vi "Image scale.vi"(2 "Error in":errorcluster, 3 "Scale factor":dbl=1.0, 4 "Image in":T1) -> (0 "Error Out":errorcluster, 1 "Image Out":T1)   [LabVIEW 2014]
uses:
  <vilib>/vision/Image Controls.llb/IMAQ Image.ctl
  <vilib>/vision/NI_Vision_Development_Module.lvlib
panel:
  # "Paul Nathan 10/06/2015"
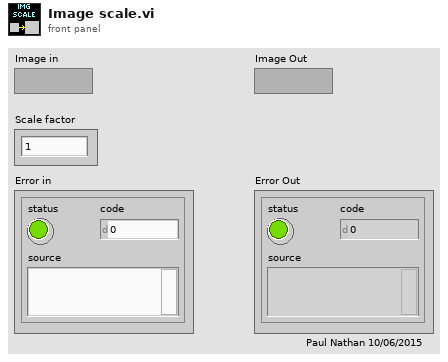
[diagram p1: front panel]
types:
  T1 = typedef "IMAQ Image.ctl" = refnum<image>
  T2 = cluster{"Red (or Hue) value":u8, "Green (or Sat) value":u8, "Blue (or Light or Val) value":u8}[][]
  T3 = cluster{"Red or Hue value":u8, "Green or Sat value":u8, "Blue or Luma or Val or Inten value":u8}
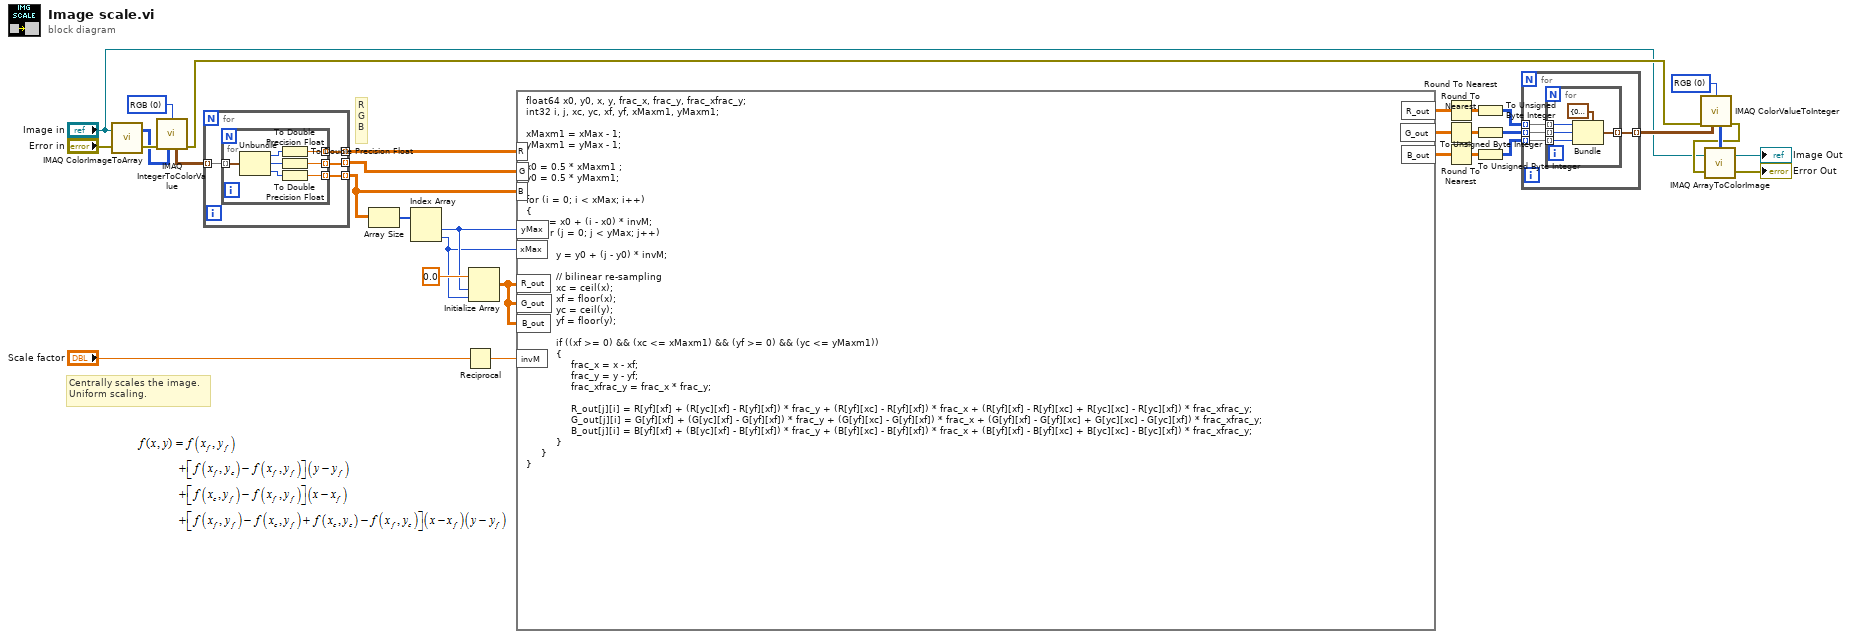
[diagram p0: block diagram]
diagram:
  w11 = u16 0 items=["RGB", "HSL", "HSV", "HSI"] ("Color Mode")
  w29 = u16 0 items=["RGB", "HSL", "HSV", "HSI"] ("Color Mode")
  # "Centrally scales the image.\nUniform scaling."
  # "R\nG\nB"
  n1 = call "IMAQ ColorImageToArray"("Image"="Image in", "error in (no error)"="Error in") -> ("Image Pixels (U32)"=w30:u32[][], "error out"=w32:errorcluster)  [unwired: 2 in, 1 out]
  n2 = call "IMAQ IntegerToColorValue"("error in (no error)"=w32, "2D U32 array"=w30, "Color Mode"=w29) -> ("2D Color value array"=w31:T2, "error out"=w7:errorcluster)  [unwired: 2 in, 2 out]
  n3 = for {
    tunnel: w31 -> [w36] mode=indexing
    tunnel: [w35] -> w27 mode=indexing
    tunnel: [w34] -> w26 mode=indexing
    tunnel: [w33] -> w24 mode=indexing
    n4 = for {
      tunnel: w36 -> [w43] mode=indexing
      tunnel: [w39] -> w35 mode=indexing
      tunnel: [w38] -> w34 mode=indexing
      tunnel: [w37] -> w33 mode=indexing
      n5 = Unbundle(w43) -> ("Red (or Hue) value"=w42:u8, "Green (or Sat) value"=w40:u8, "Blue (or Light or Val) value"=w41:u8)
      n6 = To Double Precision Float(number=w42) -> (double precision float=w39:dbl)
      n7 = To Double Precision Float(number=w40) -> (double precision float=w38:dbl)
      n8 = To Double Precision Float(number=w41) -> (double precision float=w37:dbl)
    }
  }
  n9 = Array Size(array=w24) -> (size(s)=w25:i32[])
  n10 = Index Array(array=w25) -> (element #1=w22:i32, element #2=w21:i32)  [unwired: 2 in]
  n11 = Reciprocal(x="Scale factor") -> (1/x=w1:dbl)
  n12 = Initialize Array(0.0, w22, w21) -> (w20:dbl[][])
  n13 = formula code="float64 x0, y0, x, y, frac_x, frac_y, frac_xfrac_y;\nint32 i, j, xc, yc, xf, yf, xMaxm1, yMaxm1;\n\nxMaxm1 = xMax - 1;\nyMaxm1 = yMax - 1;\n\nx0 = 0.5 * xMaxm1 ;\ny0 = 0.5 * yMaxm1; \n\nfor (i = 0; i < xMax; i++)\n{\n     x = x0 + (i - x0) * invM;\n     for (j = 0; j < yMax; j++)\n     {\n          y = y0 + (j - y0) * invM;\n          \n          // bilinear re-sampling \n          xc = ceil(x);\n          xf = floor(x);\n          yc = ceil(y);\n          yf = floor(y);\n               \n          if ((xf >= 0) && (xc <= xMaxm1) && (yf >= 0) && (yc <= yMaxm1))\n          {\n               frac_x = x - xf;\n               frac_y = y - yf;\n               frac_xfrac_y = frac_x * frac_y;\n               \n               R_out[j][i] = R[yf][xf] + (R[yc][xf] - R[yf][xf]) * frac_y + (R[yf][xc] - R[yf][xf]) * frac_x + (R[yf][xf] - R[yf][xc] + R[yc][xc] - R[yc][xf]) * frac_xfrac_y;\n               G_out[j][i] = G[yf][xf] + (G[yc][xf] - G[yf][xf]) * frac_y + (G[yf][xc] - G[yf][xf]) * frac_x + (G[yf][xf] - G[yf][xc] + G[yc][xc] - G[yc][xf]) * frac_xfrac_y;\n               B_out[j][i] = B[yf][xf] + (B[yc][xf] - B[yf][xf]) * frac_y + (B[yf][xc] - B[yf][xf]) * frac_x + (B[yf][xf] - B[yf][xc] + B[yc][xc] - B[yc][xf]) * frac_xfrac_y;\n          }\n     }\n}"("R"=w27, "G"=w26, "B"=w24, "invM"=w1, "xMax"=w21, "yMax"=w22, "R_out"=w20, "G_out"=w20, "B_out"=w20) -> ("R_out"=w10:dbl[][], "G_out"=w9:dbl[][], "B_out"=w8:dbl[][])
  n14 = Round To Nearest(number=w10) -> (nearest integer value=w12:dbl[][])
  n15 = Round To Nearest(number=w9) -> (nearest integer value=w13:dbl[][])
  n16 = Round To Nearest(number=w8) -> (nearest integer value=w14:dbl[][])
  n17 = To Unsigned Byte Integer(number=w12) -> (unsigned 8bit integer=w17:u8[][])
  n18 = To Unsigned Byte Integer(number=w13) -> (unsigned 8bit integer=w16:u8[][])
  n19 = To Unsigned Byte Integer(number=w14) -> (unsigned 8bit integer=w15:u8[][])
  n20 = for {
    tunnel: w15 -> [w47] mode=indexing
    tunnel: w16 -> [w46] mode=indexing
    tunnel: w17 -> [w45] mode=indexing
    tunnel: [w44] -> w18 mode=indexing
    n21 = for {
      tunnel: w47 -> [w51] mode=indexing
      tunnel: w46 -> [w50] mode=indexing
      tunnel: w45 -> [w49] mode=indexing
      tunnel: [w48] -> w44 mode=indexing
      n22 = Bundle(cluster=T3 {"Red or Hue value"=0, "Green or Sat value"=0, "Blue or Luma or Val or Inten value"=0} ("Color Value"), "Red or Hue value"=w49, "Green or Sat value"=w50, "Blue or Luma or Val or Inten value"=w51) -> (w48:T3)
    }
  }
  n23 = call "IMAQ ColorValueToInteger"("error in (no error)"=w7, "2D Color value array"=w18, "Color Mode"=w11) -> ("2D U32 array"=w19:u32[][], "error out"=w6:errorcluster)  [unwired: 2 in, 2 out]
  n24 = call "IMAQ ArrayToColorImage"("Image Pixels (U32)"=w19, "Image"="Image in", "error in (no error)"=w6) -> ("Image Out"=→"Image Out":T1, "error out"=→"Error Out":errorcluster)  [unwired: 2 in]
